vi "tcs shm get Sample kernel Pointing Log LV.vi"(8 "error in (no error)":errorcluster, 11 "kernel_PointingLog_Ctl":T1) -> (0 "error out":errorcluster, 2 "function return":i32, 3 "kernel_PointingLog_Ctl out":T1)   [LabVIEW 2016, in "SALLV_tcs.lvlib"]
doc: "int tcs_shm_getSample_kernel_PointingLogLV(tcs_kernel_PointingLogLV *kernel_PointingLog_Ctl );"
uses:
  SALLV_tcs.lvlib
  SALLV_tcs.so
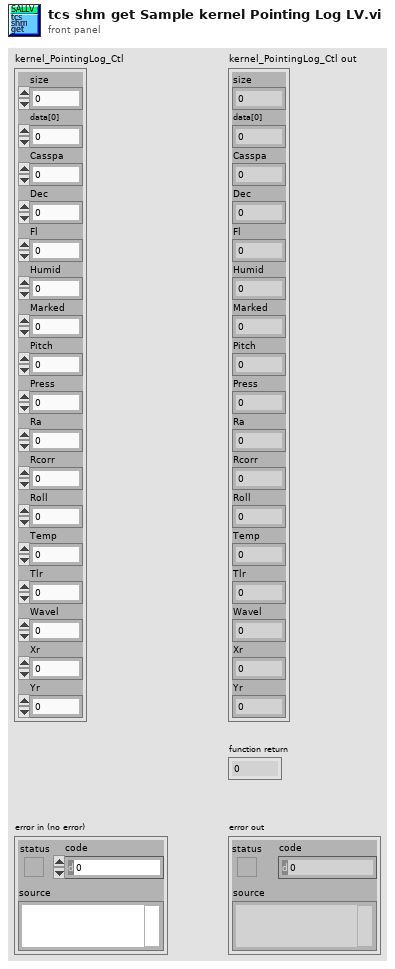
[diagram p1: front panel]
types:
  T1 = cluster{"size":i32, "data[0]":sgl, "Casspa":sgl, "Dec":sgl, "Fl":sgl, "Humid":sgl, "Marked":i32, "Pitch":sgl, "Press":sgl, "Ra":sgl, "Rcorr":sgl, "Roll":sgl, "Temp":sgl, "Tlr":sgl, "Wavel":sgl, "Xr":sgl, "Yr":sgl}
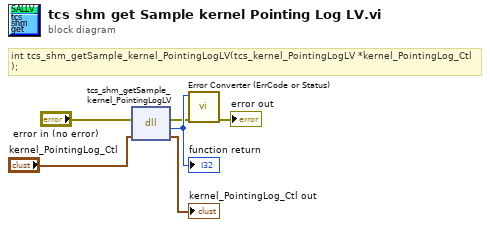
[diagram p0: block diagram]
diagram:
  # "int tcs_shm_getSample_kernel_PointingLogLV(tcs_kernel_PointingLogLV *kernel_PointingLog_Ctl );"
  n1 = dll-call lib="home/andres/Desktop/SALLV_tcs/SALLV_tcs.*" fn="tcs_shm_getSample_kernel_PointingLogLV"(error in="error in (no error)", "kernel_PointingLog_Ctl"="kernel_PointingLog_Ctl") -> (error out=w2:errorcluster, w6:i32, "kernel_PointingLog_Ctl"=→"kernel_PointingLog_Ctl out":T1)  [unwired: 2 in, 1 out]
  "function return" <- w6
  n2 = call "Error Converter (ErrCode or Status).vi"("error in (no error)"=w2, "error code"=w6) -> ("error out"=→"error out":errorcluster)  [unwired: 9 in]
